vi "read_string.vi"(8 "error in":errorcluster, 11 "VISA resource name":refnum<visa-resource-name>) -> (0 "error out":errorcluster, 2 "read buffer":string, 3 "VISA resource name out":refnum<visa-resource-name>)   [LabVIEW 2016]
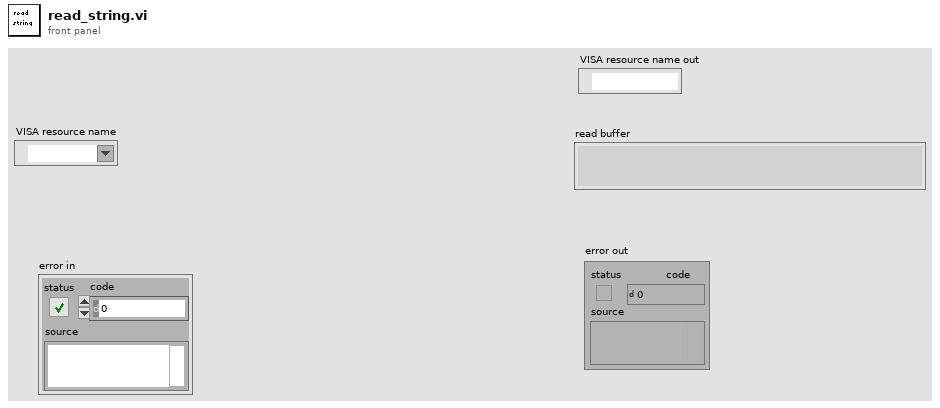
[diagram p1: front panel]
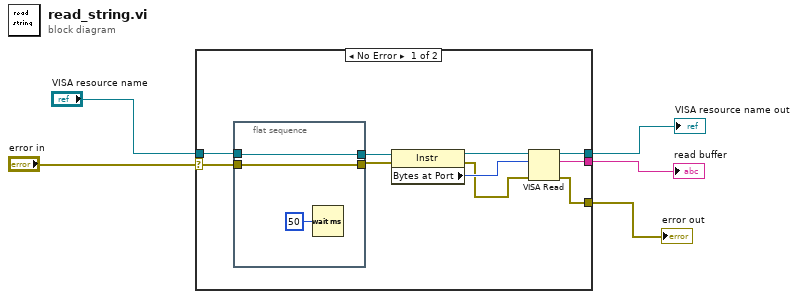
[diagram p0: block diagram]
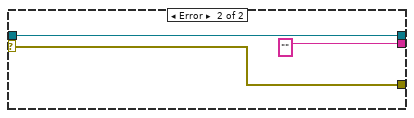
[diagram p2: hidden frame]
diagram:
  n1 = case shown="No Error" "error in" {
    selector: "error in" -> [w6 w21]
    tunnel: "VISA resource name" -> [w9 w19]
    tunnel: [w15 "" ("read buffer")] -> w5
    tunnel: [w14 w19] -> w4
    tunnel: [w13 w21] -> w2
    frame No Error {
      n2 = flat-sequence {
        tunnel: [w17] -> w8
        tunnel: w9 -> [w17]
        tunnel: [w16] -> w7
        tunnel: w6 -> [w16]
        frame #0 {
          n3 = Wait (ms)(milliseconds to wait=u32 50 ("millisecond multiple")) -> ()  [unwired: 1 out]
        }
      }
      n4 = property class="Instr"(reference=w8, error in=w7) -> (reference out=w11:refnum<visa-resource-name>, error out=w10:errorcluster, "Bytes at Port"=w12:u32)
      n5 = VISA Read(VISA resource name=w11, byte count=w12, error in (no error)=w10) -> (VISA resource name out=w14:refnum<visa-resource-name>, read buffer=w15:string, error out=w13:errorcluster)  [unwired: 1 out]
    }
    frame Error {
    }
  }
  "read buffer" <- w5
  "VISA resource name out" <- w4
  "error out" <- w2
